vi "saltso prueba.vi"() -> ()   [LabVIEW 2010]
uses:
  <vilib>/vision/Image Controls.llb/IMAQ Image.ctl
panel:
  out "Tomando Saltos":bool=TRUE
  out "Estable":bool=TRUE
  in  "Path":path
  out "appended path":path
  out "Freq Output":dbl
  in  "Image Device IN":cluster{"Image":T1, "errorImage":errorcluster}
  in  "Comienza Saltos":bool=TRUE
  in  "Parametros de Saltos":T2
  in  "stop":bool
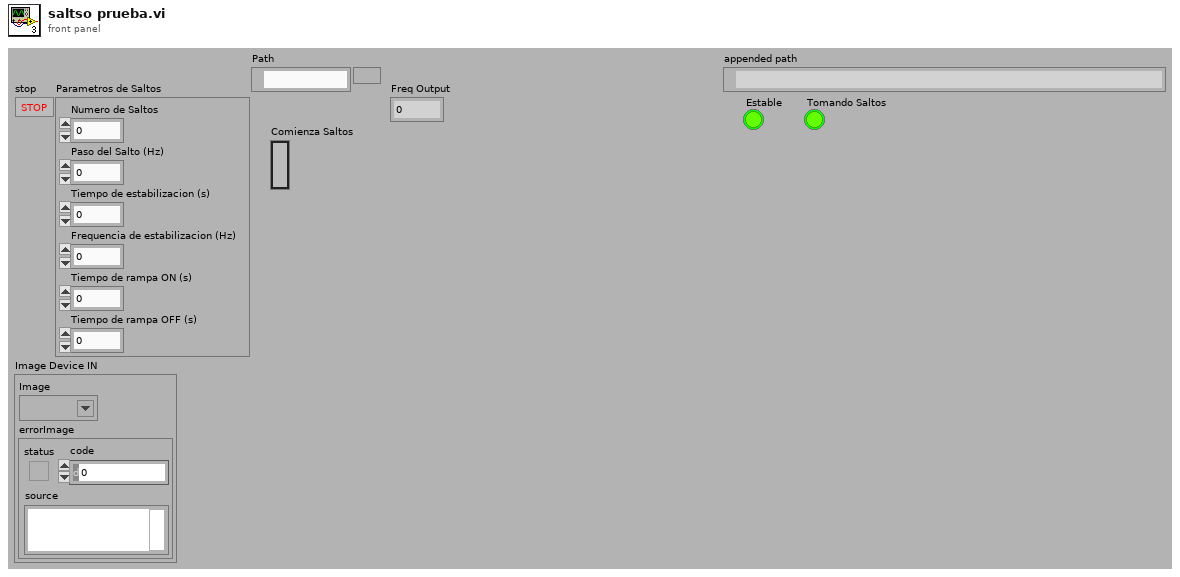
[diagram p1: front panel]
types:
  T1 = typedef "IMAQ Image.ctl" = refnum<image>
  T2 = cluster{"Numero de Saltos":i32, "Paso del Salto (Hz)":dbl, "Tiempo de estabilizacion (s)":dbl, "Frequencia de estabilizacion (Hz)":dbl, "Tiempo de rampa ON (s)":dbl, "Tiempo de rampa OFF (s)":dbl}
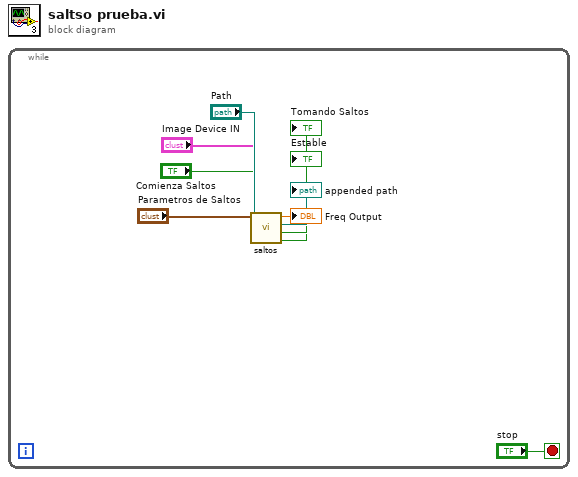
[diagram p0: block diagram]
diagram:
  n1 = while {
    stop <- "stop" stop-if-true
    n2 = call "saltos.vi"("Image Device IN"="Image Device IN", "Comienza Saltos"="Comienza Saltos", "Path"="Path", "Parametros de Saltos"="Parametros de Saltos") -> ("Tomando Saltos"=→"Tomando Saltos":bool, "Estable"=→"Estable":bool, "appended path"=→"appended path":path, "Freq Output"=→"Freq Output":dbl)  [unwired: 4 in]
  }
